vi "acq_eeg_ini.vi"(8 "error in (no error)":errorcluster, 11 "eeg_device in":T1) -> (0 "error out":errorcluster, 2 "Variant":variant)   [LabVIEW 2013]
doc: "Opens the communication with the EEG device, based on its hardware"
uses:
  <vilib>/NIOSC/Address Space Node.ctl
  gui/type_def/device.ctl
  <vilib>/OpenBCI/Comm Protocol/Control Def/channel_count.ctl
  gui/type_def/file_stream.ctl
  gui/global_var.vi
  <vilib>/NI/Emotiv Toolkit/Emotiv Create Task Instances/EmoEngine.vi
  <vilib>/NI/Emotiv Toolkit/Emotiv Start Task Instances/Basic Start Task.vi
  <vilib>/NIOSC/NI_OSC.lvlib
  <vilib>/NI/Emotiv Toolkit/Emotiv Task.lvclass
  <vilib>/NI/LabVIEW - NeuroSky Driver/NeuroSky Driver.lvlib
panel:
  in  "muse cluster":T3
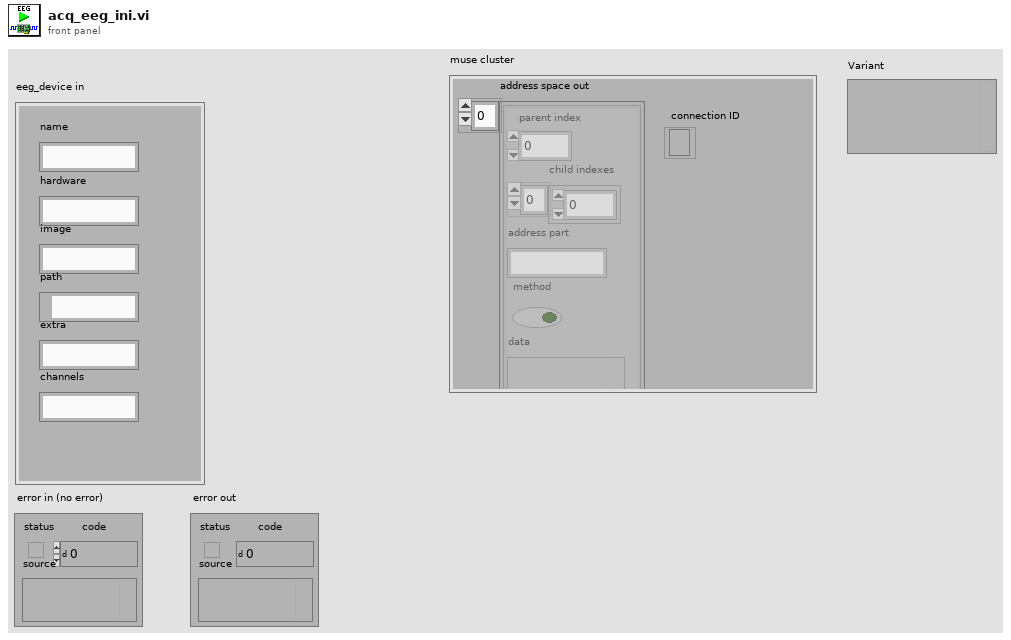
[diagram p1: front panel]
types:
  T1 = typedef "device.ctl" = cluster{"name":string, "hardware":string, "image":string, "path":path, "extra":string, "channels":string}
  T2 = typedef "NI_OSC.lvlib/Address Space Node.ctl" = cluster{"parent index":i32, "child indexes":i32[], "address part":string, "method":bool, "data":variant}
  T3 = cluster{"address space out":T2[], "connection ID":refnum<k5>}
  T4 = typedef "channel_count.ctl" = enum16{"8 Channels", "16 Channels"}
  T5 = typedef "file_stream.ctl" = cluster{"timestamp":timestamp, "data (2D array)":dbl[][], "Reading?":bool}
  T6 = cluster{"connectionId":i32, "serialPortName":string, "serialBaudrate":i32, "serialDataFormat":i32}
  T7 = typedef "openbci_device.ctl" = cluster{"COM port":refnum<visa-resource-name>, "n_ch (8)":T4, "delay_tx":u32}
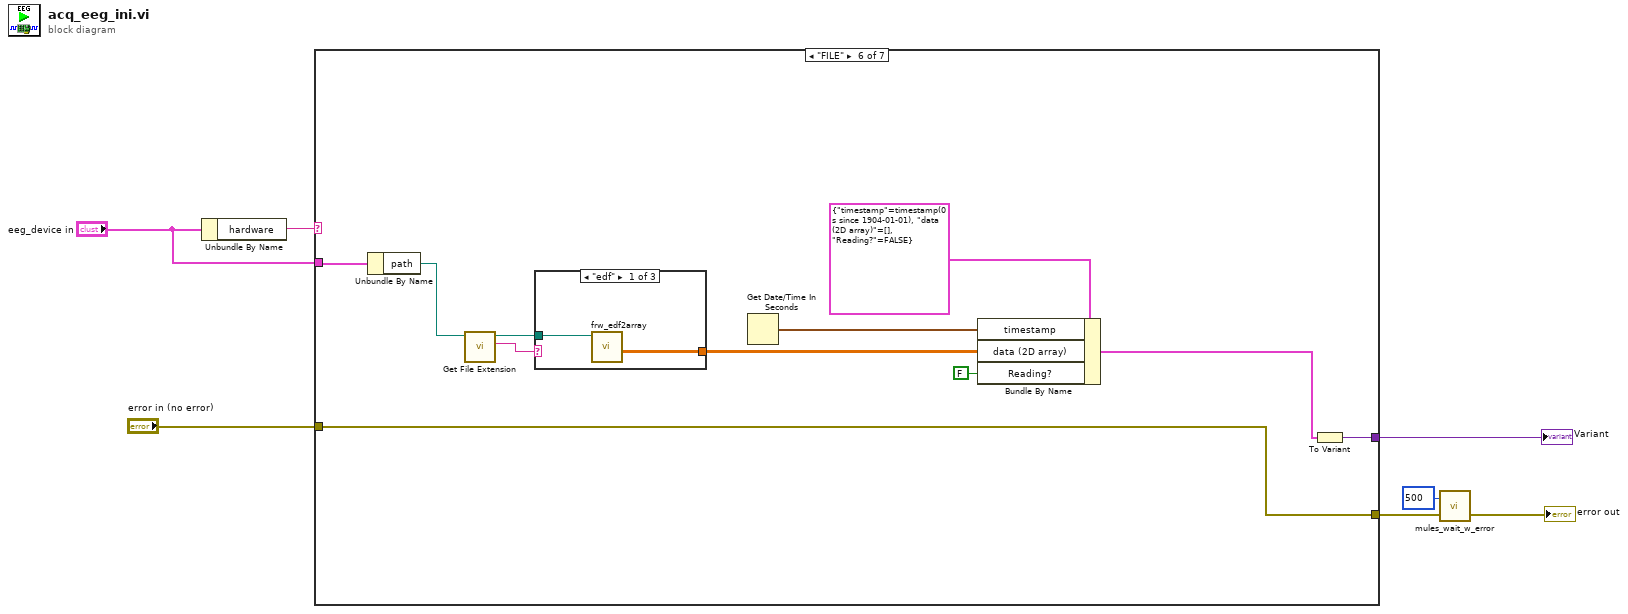
[diagram p0: block diagram]
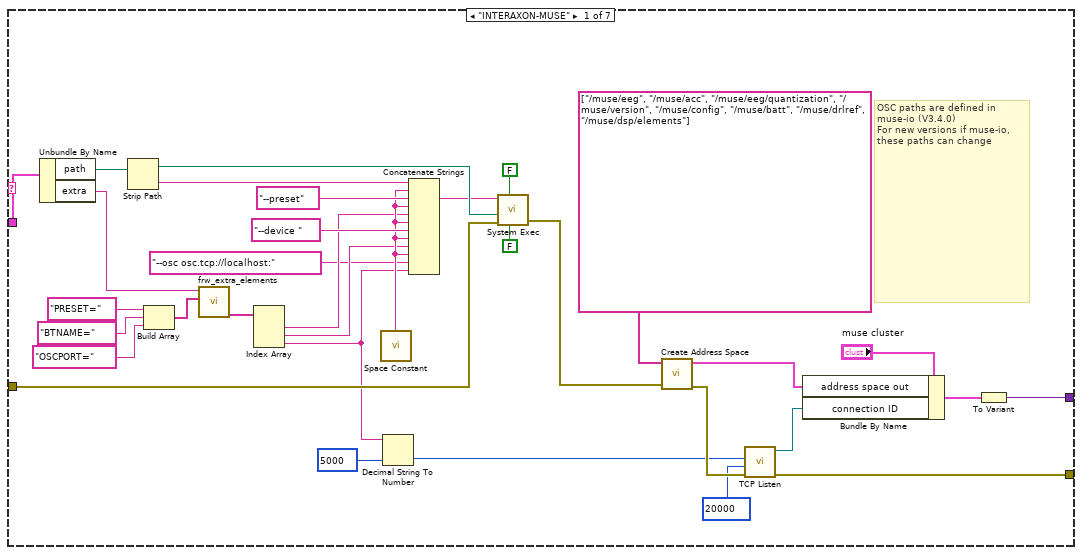
[diagram p2: hidden frame]
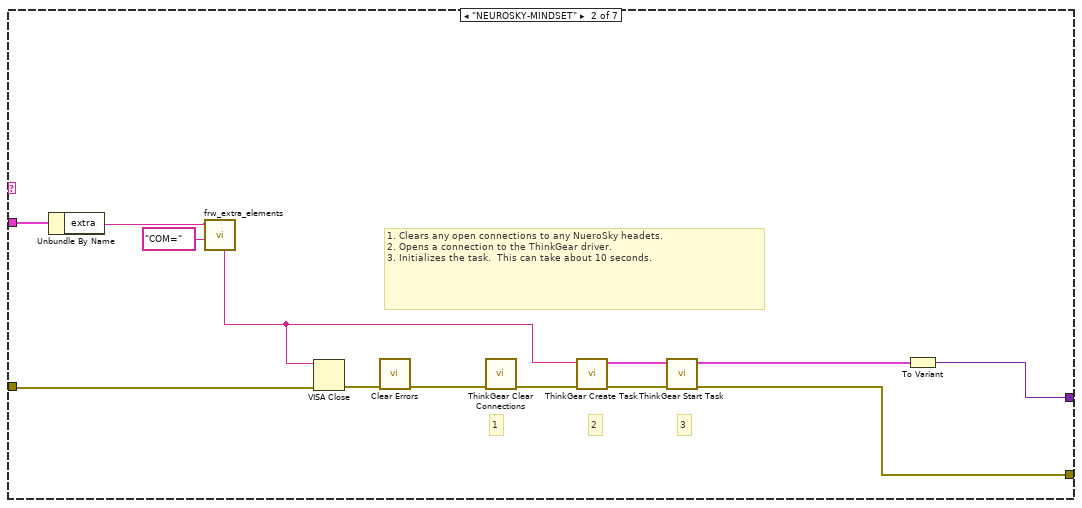
[diagram p3: hidden frame]
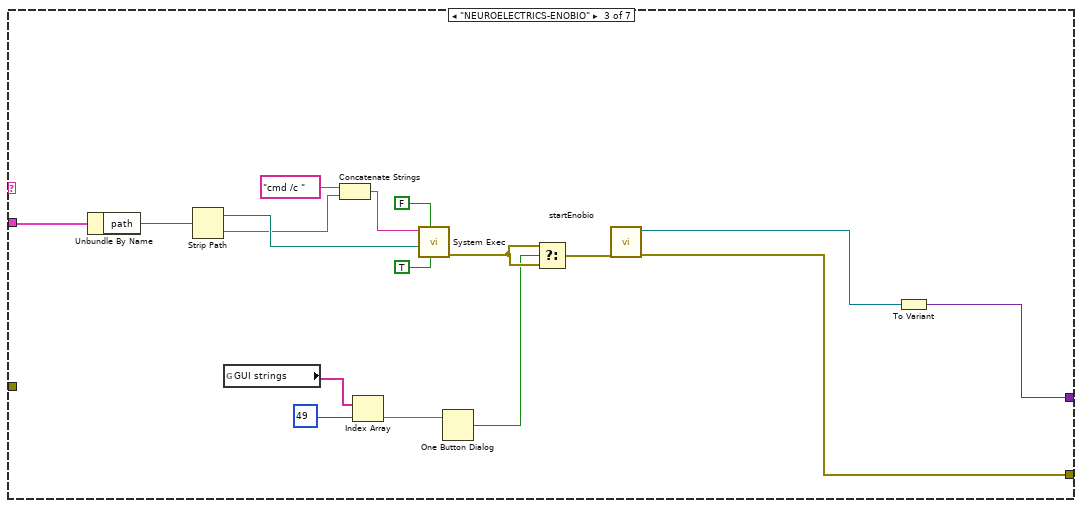
[diagram p4: hidden frame]
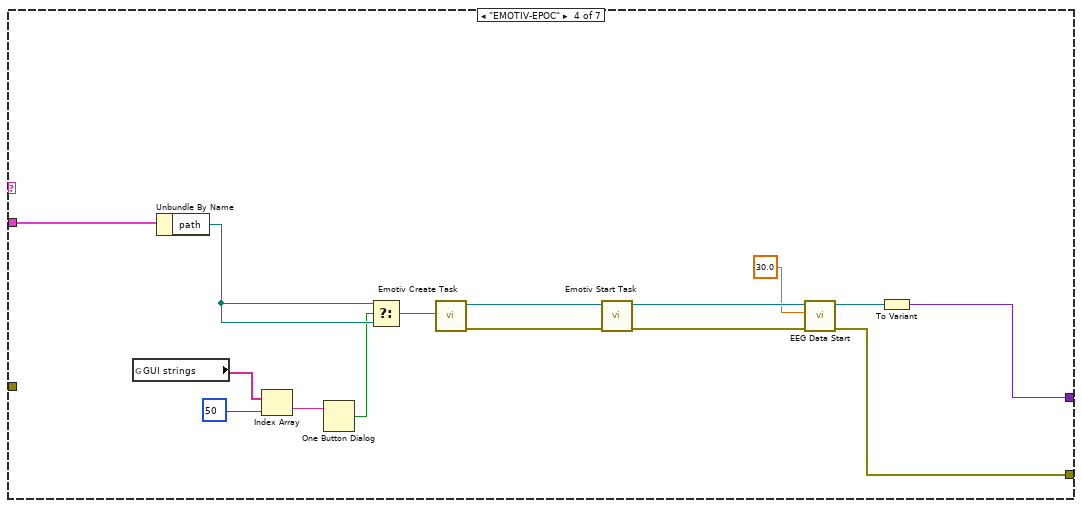
[diagram p5: hidden frame]
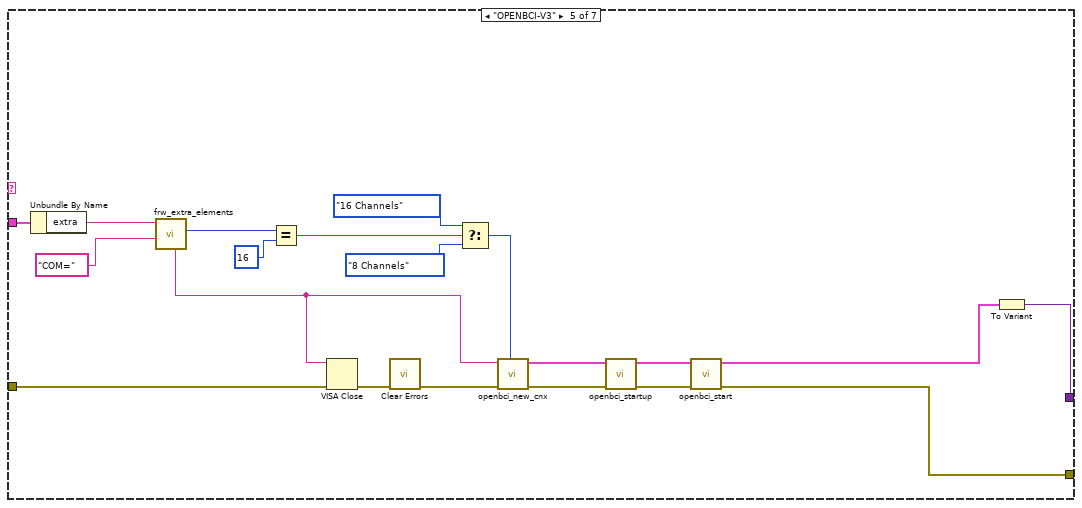
[diagram p6: hidden frame]
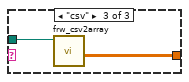
[diagram p8: hidden frame]
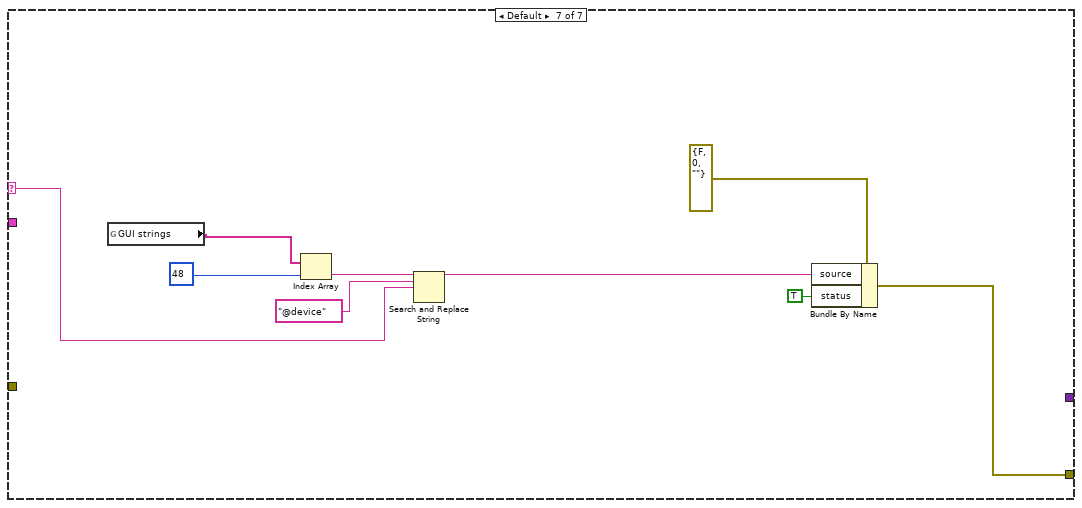
[diagram p9: hidden frame]
diagram:
  n1 = Unbundle By Name("eeg_device in") -> ("hardware"=w7:string)
  n2 = case shown="\"FILE\"" w7 {
    selector: w7 -> [_ _ _ _ _ _ w125]
    tunnel: "eeg_device in" -> [w40 w50 w70 w85 w105 w114 _]
    tunnel: "error in (no error)" -> [w36 w45 _ _ w98 w116 _]
    tunnel: [w27 w49 w64 w79 w96 w116 w123] -> w4
    tunnel: [w35 w48 w66 w78 w101 w108 _] -> w5
    frame "INTERAXON-MUSE" {
      # "OSC paths are defined in muse-io (V3.4.0)\nFor new versions if muse-io, these paths can change"
      n3 = Unbundle By Name(w40) -> ("path"=w39:path, "extra"=w13:string)
      n4 = Strip Path(path=w39) -> (stripped path=w38:path, name=w24:string)
      n5 = Build Array("PRESET=" ("delimiter (Tab)"), "BTNAME=" ("delimiter (Tab)"), "OSCPORT=" ("delimiter (Tab)")) -> (w17:string[])
      n6 = call "frw_extra_elements.vi"("fields"=w17, "string"=w13) -> ("values"=w12:string[])  [unwired: 5 in, 4 out]
      n7 = Index Array(array=w12) -> (element #1=w11:string, element #2=w10:string, element #3=w8:string)  [unwired: 3 in]
      n8 = call <vilib>:"Space Constant.vi"() -> ("String"=w18:string)
      n9 = Decimal String To Number(string=w8, default (0L)=u16 5000 ("Local Port")) -> (number=w23:u16)  [unwired: 1 in, 1 out]
      n10 = Concatenate Strings(w24, w18, "--preset" ("string"), w18, w11, w18, "--device " ("string"), w18, w10, w18, "--osc osc.tcp://localhost:" ("string"), w8) -> (w26:string)
      n11 = call <vilib>:"System Exec.vi"("run minimized? (F)"=FALSE, "wait until completion? (T)"=FALSE, "error in (no error)"=w36, "working directory"=w38, "command line"=w26) -> ("error out"=w32:errorcluster)  [unwired: 3 in, 3 out]
      n12 = call <vilib>:"Create Address Space.vi"("error in"=w32, "method addresses"=string[] ["/muse/eeg", "/muse/acc", "/muse/eeg/quantization", "/muse/version", "/muse/config", "/muse/batt", "/muse/drlref", "/muse/dsp/elements"]) -> ("error out"=w33:errorcluster, "address space out"=w30:T2[])  [unwired: 8 in]
      n13 = call <vilib>:"TCP Listen.vi"("error in (no error)"=w33, "timeout ms (wait forever: -1)"=20000, "port"=w23) -> ("error out"=w27:errorcluster, "connection ID"=w29:refnum<k5>)  [unwired: 4 in, 3 out]
      n14 = Bundle By Name(cluster="muse cluster", "address space out"=w30, "connection ID"=w29) -> (w28:T3)
      n15 = To Variant(anything=w28) -> (Variant=w35:variant)
    }
    frame "NEUROSKY-MINDSET" {
      # "1. Clears any open connections to any NueroSky headets.\n2. Opens a connection to the ThinkGear driver.\n3. Initializes the task.  This can take about 10 seconds."
      # "1"
      # "3"
      # "2"
      n16 = Unbundle By Name(w50) -> ("extra"=w43:string)
      n17 = call "frw_extra_elements.vi"("single field"="COM=", "string"=w43) -> ("single string"=w41:string)  [unwired: 5 in, 4 out]
      n18 = VISA Close(VISA resource name=w41, error in (no error)=w45) -> (error out=w46:errorcluster)
      n19 = call <vilib>:"Clear Errors.vi"("error in (no error)"=w46) -> ("error out"=w44:errorcluster)  [unwired: 6 in]
      n20 = call <vilib>:"ThinkGear Clear Connections.vi"("error in (no error)"=w44) -> ("error out"=w51:errorcluster)  [unwired: 10 in]
      n21 = call <vilib>:"ThinkGear Create Task.vi"("error in"=w51, "serialPortName"=w41) -> ("error out"=w52:errorcluster, "NeuroSky Task Out"=w53:T6)  [unwired: 8 in]
      n22 = call <vilib>:"ThinkGear Start Task.vi"("error in (no error)"=w52, "NeuroSky Task In"=w53) -> ("error out"=w49:errorcluster, "NeuroSky Task Out"=w47:T6)  [unwired: 8 in]
      n23 = To Variant(anything=w47) -> (Variant=w48:variant)
    }
    frame "NEUROELECTRICS-ENOBIO" {
      n24 = Unbundle By Name(w70) -> ("path"=w69:path)
      n25 = Strip Path(path=w69) -> (stripped path=w68:path, name=w59:string)
      n26 = global read "global_var.vi" "GUI strings"() -> (w56:string[])
      n27 = Concatenate Strings("cmd /c " ("string"), w59) -> (w58:string)
      n28 = Index Array(array=w56, index=49) -> (element=w54:string)
      n29 = call <vilib>:"System Exec.vi"("run minimized? (F)"=TRUE, "wait until completion? (T)"=FALSE, "working directory"=w68, "command line"=w58) -> ("error out"=w62:errorcluster)  [unwired: 4 in, 3 out]
      n30 = One Button Dialog(message=w54) -> (true=w61:bool)  [unwired: 1 in]
      n31 = Select(t=w62, s=w61, f=w62) -> (s? t:f=w63:errorcluster)
      n32 = call "startEnobio.vi"("error in (no error)"=w63) -> ("error out"=w64:errorcluster, "connection ID"=w65:refnum<k5>)  [unwired: 9 in]
      n33 = To Variant(anything=w65) -> (Variant=w66:variant)
    }
    frame "EMOTIV-EPOC" {
      n34 = global read "global_var.vi" "GUI strings"() -> (w73:string[])
      n35 = Unbundle By Name(w85) -> ("path"=w75:path)
      n36 = Index Array(array=w73, index=50) -> (element=w71:string)
      n37 = One Button Dialog(message=w71) -> (true=w74:bool)  [unwired: 1 in]
      n38 = Select(t=w75, s=w74, f=w75) -> (s? t:f=w76:path)
      n39 = call-poly <vilib>:"Emotiv Create Task.vi"("edk.dll Path"=w76) -> ("error out"=w84:errorcluster, "Emotiv Task out"=w83:refnum<class "Emotiv Task.lvclass">)  [unwired: 9 in]
      n40 = call-poly <vilib>:"Emotiv Start Task.vi"("error in (no error)"=w84, "Emotiv Task in"=w83) -> ("error out"=w82:errorcluster, "Emotiv Task out"=w81:refnum<class "Emotiv Task.lvclass">)  [unwired: 6 in]
      n41 = call <vilib>:"EEG Data Start.vi"("error in (no error)"=w82, "bufferSizeInSec"=sgl 30.0 ("BufferSize Emotive (sec)"), "Emotiv Task in"=w81) -> ("error out"=w79:errorcluster, "Emotiv Task out"=w77:refnum<class "Emotiv Task.lvclass">)  [unwired: 7 in]
      n42 = To Variant(anything=w77) -> (Variant=w78:variant)
    }
    frame "OPENBCI-V3" {
      n43 = Unbundle By Name(w105) -> ("extra"=w91:string)
      n44 = call "frw_extra_elements.vi"("single field"="COM=" ("delimiter (Tab)"), "string"=w91) -> ("fs"=w90:i32, "single string"=w86:string)  [unwired: 5 in, 3 out]
      n45 = Equal?(x=w90, y=16) -> (x = y?=w88:bool)
      n46 = VISA Close(VISA resource name=w86, error in (no error)=w98) -> (error out=w93:errorcluster)
      n47 = call <vilib>:"Clear Errors.vi"("error in (no error)"=w93) -> ("error out"=w92:errorcluster)  [unwired: 6 in]
      n48 = Select(t=channel_count."16 Channels" ("channel_count(8)"), s=w88, f=channel_count."8 Channels" ("channel_count(8)")) -> (s? t:f=w102:T4)
      n49 = call <vilib>:"openbci_new_cnx.vi"("channel_count(8)"=w102, "error in (no error)"=w92, "COM port"=w86) -> ("error out"=w99:errorcluster, "OBCI dev out"=w100:T7)  [unwired: 7 in]
      n50 = call <vilib>:"openbci_startup.vi"("error in"=w99, "OBCI dev in"=w100) -> ("error out"=w97:errorcluster, "OBCI dev out"=w95:T7)  [unwired: 7 in, 1 out]
      n51 = call <vilib>:"openbci_start.vi"("error in (no error)"=w97, "OBCI dev in"=w95) -> ("error out"=w96:errorcluster, "OBCI dev out"=w94:T7)  [unwired: 8 in]
      n52 = To Variant(anything=w94) -> (Variant=w101:variant)
    }
    frame "FILE" {
      n53 = Unbundle By Name(w114) -> ("path"=w110:path)
      n54 = call <vilib>:"Get File Extension.vi"("file"=w110) -> ("lowercase file extension"=w115:string, "dup file"=w109:path)  [unwired: 7 in, 2 out]
      n55 = case shown="\"edf\"" w115 {
        tunnel: w109 -> [w118 _ w120]
        tunnel: [w117 _ w119] -> w111
        frame "edf" {
          n56 = call "frw_edf2array.vi"("file path"=w118) -> ("2D array"=w117:dbl[][])  [unwired: 8 in, 2 out]
        }
        frame Default {
        }
        frame "csv" {
          n57 = call "frw_csv2array.vi"("file path"=w120) -> ("values"=w119:dbl[][])  [unwired: 7 in, 3 out]
        }
      }
      n58 = Get Date/Time In Seconds() -> (seconds since 1Jan1904=w112:timestamp)
      n59 = Bundle By Name(cluster=T5 {"timestamp"=timestamp(0 s since 1904-01-01), "data (2D array)"=[], "Reading?"=FALSE} ("output cluster"), "timestamp"=w112, "data (2D array)"=w111, "Reading?"=FALSE) -> (w107:T5)
      n60 = To Variant(anything=w107) -> (Variant=w108:variant)
    }
    frame Default {
      n61 = global read "global_var.vi" "GUI strings"() -> (w127:string[])
      n62 = Index Array(array=w127, index=48) -> (element=w128:string)
      n63 = Search and Replace String(input string=w128, search string="@device", replace string=w125) -> (result string=w122:string)  [unwired: 5 in, 3 out]
      n64 = Bundle By Name(cluster=errorcluster {"status"=FALSE, "code"=0, "source"=""} ("error constant"), "source"=w122, "status"=TRUE) -> (w123:errorcluster)
    }
  }
  "Variant" <- w5
  n65 = call "mules_wait_w_error.vi"("error in (no error)"=w4, "milliseconds to wait"=u32 500) -> ("error out"=→"error out":errorcluster)  [unwired: 1 in]
